vi "Freq_Seperate_Z.vi"(0 "constraint":dbl[](array[numeric]), 1 "Length":i32) -> (3 "weight":dbl, 4 "alpha":dbl, 5 "beta":dbl[](array[numeric]), 6 "gamma":dbl, 7 "Omega":dbl[][](array[numeric]))   [LabVIEW 2015]
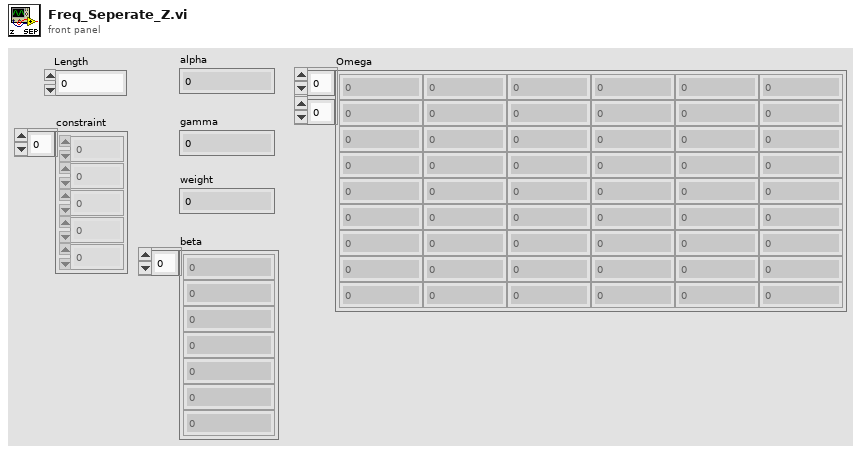
[diagram p1: front panel]
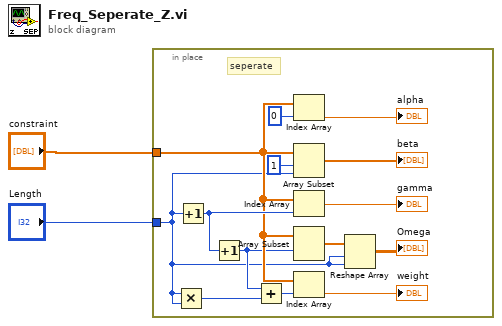
[diagram p0: block diagram]
diagram:
  n1 = in-place {
    in-place-border: "constraint" -> [w9]
    in-place-border: "Length" -> [w6]
    # "seperate"
    n2 = Multiply(x=w6, y=w6) -> (x*y=w5:i32)
    n3 = Increment(x=w6) -> (x+1=w14:i32)
    n4 = Increment(x=w14) -> (x+1=w7:i32)
    n5 = Add(x=w7, y=w5) -> (x+y=w8:i32)
    n6 = Index Array(array=w9, index=0) -> (element=→"alpha":dbl)
    n7 = Array Subset(array=w9, index=1, length=w6) -> (→"beta":dbl[])
    n8 = Index Array(array=w9, index=w14) -> (element=→"gamma":dbl)
    n9 = Array Subset(array=w9, index=w7) -> (w13:dbl[])  [unwired: 1 in]
    n10 = Index Array(array=w9, index=w8) -> (element=→"weight":dbl)
    n11 = Reshape Array(w13, w6, w6) -> (→"Omega":dbl[][])
  }
